vi "GT Get Axis Prf Vel Filter.vi"(8 "error in (no error)":errorcluster caption="错误输入（无错误）", 9 "pFilterNumExp":i16[](array[numeric]), 10 "axis":i16, 11 "cardNum":i16) -> (0 "error out":errorcluster caption="错误输出", 1 "pFilterNumExp out":i16[](array[numeric]), 3 "function return":i16)   [LabVIEW 2020, in "gts.lvlib"]
doc: "GT_API GT_GetAxisPrfVelFilter(short cardNum,short axis,short *pFilterNumExp);"
uses:
  gts.lvlib
  dll/32bit/multi_card/gts.dll
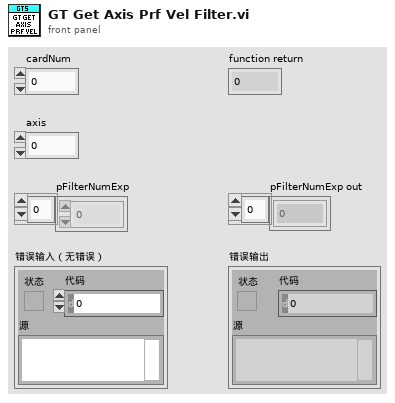
[diagram p1: front panel]
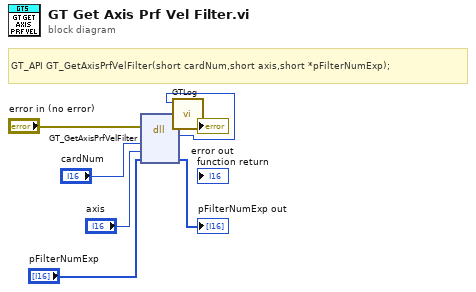
[diagram p0: block diagram]
diagram:
  # "GT_API GT_GetAxisPrfVelFilter(short cardNum,short axis,short *pFilterNumExp);"
  n1 = dll-call lib="C:/1228/dll/32bit/multi_card/gts.dll" fn="GT_GetAxisPrfVelFilter"(error in="error in (no error)", "cardNum"="cardNum", "axis"="axis", "pFilterNumExp"="pFilterNumExp") -> (error out=w3:errorcluster, "返回类型"=w1:i16, "pFilterNumExp"=→"pFilterNumExp out":i16[])  [unwired: 4 in, 1 out]
  n2 = call "GTLog.vi"("error in (no error)"=w3, "Numeric"=w1) -> ("error out"=→"error out":errorcluster)  [unwired: 9 in]
